vi "Problem2.8.vi"() -> ()   [LabVIEW 2019]
panel:
  out "Rate Limited Output":dbl
  out "Joystick Input":dbl
  in  "Rate Limit":dbl min=0.0 max=1.0 step=0.01 format="%#_2f"
  in  "Joystick Input":dbl(slide) scale=-1.0..1.0
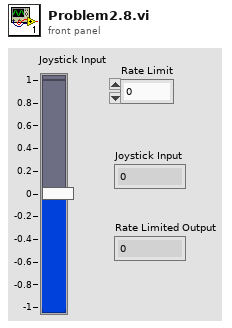
[diagram p1: front panel]
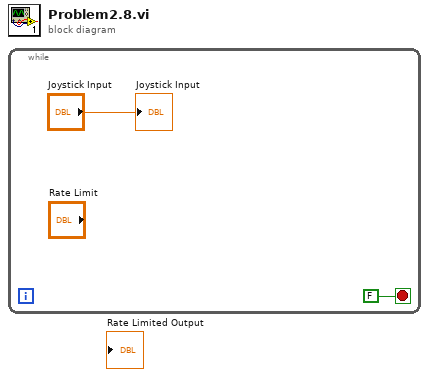
[diagram p0: block diagram]
diagram:
  n1 = while {
    stop <- FALSE stop-if-true
    "Joystick Input" <- "Joystick Input"
  }
